vi "F1_Read_Config.vi"(4 "error in (no error)":errorcluster, 7 "Config Refnum":T1) -> (0 "error out":errorcluster, 2 "All Found?":bool, 3 "refnum out":T1)   [LabVIEW 2015]
uses:
  <vilib>/Utility/config.llb/Config Data RefNum.ctl
  <vilib>/Utility/config.llb/Read Key (I32).vi
  GSP_F1_Global.vi
  <vilib>/Utility/config.llb/Read Key (Double).vi
  <vilib>/Utility/config.llb/NI_LVConfig.lvlib
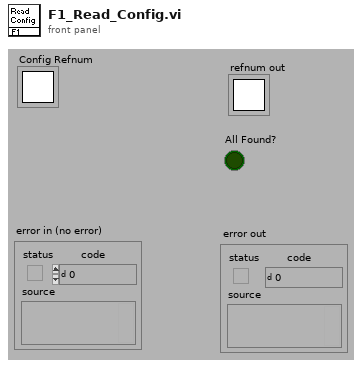
[diagram p1: front panel]
types:
  T1 = typedef "NI_LVConfig.lvlib/Config Data RefNum.ctl" = refnum<k1>
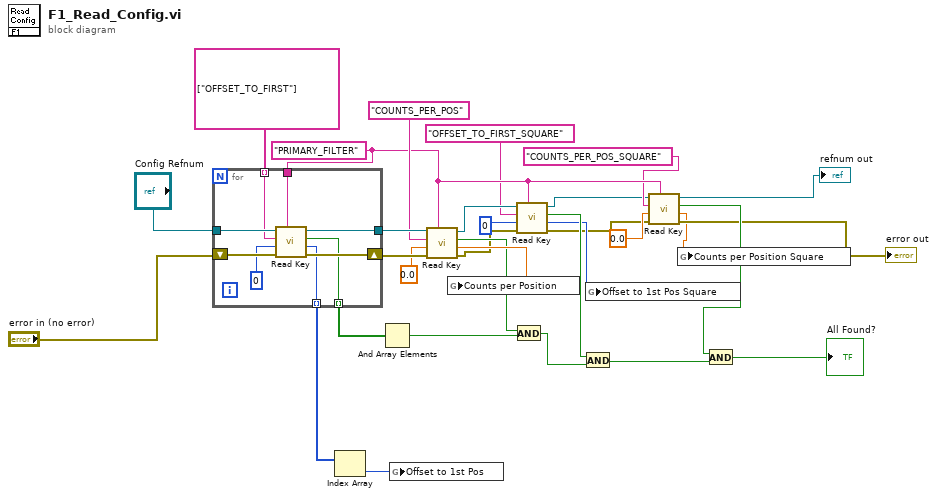
[diagram p0: block diagram]
diagram:
  w16 = "PRIMARY_FILTER"
  n1 = for {
    tunnel: "Config Refnum" -> [w39]
    shift-right: [w38] -> w27
    shift-left: "error in (no error)" -> [w40]
    tunnel: [w37] -> w28
    tunnel: string[] ["OFFSET_TO_FIRST"] -> [w36] mode=indexing
    tunnel: w16 -> [w35]
    tunnel: [w34] -> w23 mode=indexing
    tunnel: [w33] -> w22 mode=indexing
    n2 = call-poly <vilib>:"Read Key.vi"("section"=w35, "error in (no error)"=w40, "default value"=0, "key"=w36, "refnum"=w39) -> ("error out"=w38:errorcluster, "value"=w34:i32, "found?"=w33:bool, "refnum out"=w37:T1)  [unwired: 3 in]
  }
  n3 = Index Array(array=w23) -> (element=w19:i32)  [unwired: 1 in]
  n4 = And Array Elements(Boolean array=w22) -> (logical AND=w21:bool)
  n5 = global write "GSP_F1_Global.vi" "Offset to 1st Pos"(w19) -> ()
  n6 = call-poly <vilib>:"Read Key.vi"("section"=w16, "error in (no error)"=w27, "default value"=0.0, "key"="COUNTS_PER_POS", "refnum"=w28) -> ("error out"=w17:errorcluster, "value"=w24:dbl, "found?"=w20:bool, "refnum out"=w18:T1)  [unwired: 3 in]
  n7 = global write "GSP_F1_Global.vi" "Counts per Position"(w24) -> ()
  n8 = And(x=w20, y=w21) -> (x .and. y?=w15:bool)
  n9 = call-poly <vilib>:"Read Key.vi"("section"=w16, "error in (no error)"=w17, "default value"=0, "key"="OFFSET_TO_FIRST_SQUARE", "refnum"=w18) -> ("error out"=w5:errorcluster, "value"=w10:i32, "found?"=w14:bool, "refnum out"=w1:T1)  [unwired: 3 in]
  n10 = And(x=w14, y=w15) -> (x .and. y?=w13:bool)
  n11 = global write "GSP_F1_Global.vi" "Offset to 1st Pos Square"(w10) -> ()
  n12 = call-poly <vilib>:"Read Key.vi"("section"=w16, "error in (no error)"=w5, "default value"=0.0, "key"="COUNTS_PER_POS_SQUARE", "refnum"=w1) -> ("error out"=→"error out":errorcluster, "value"=w3:dbl, "found?"=w12:bool, "refnum out"=→"refnum out":T1)  [unwired: 3 in]
  n13 = global write "GSP_F1_Global.vi" "Counts per Position Square"(w3) -> ()
  n14 = And(x=w12, y=w13) -> (x .and. y?=→"All Found?":bool)
